vi "NIMS_DF_fir_linfconstr(n, f, mag, ftype, t).vi"(6 "t":enum32{"sym", "antisym", "minphase", "maxphase"}(ring), 8 "ftype":string, 9 "mag":dbl[](array[numeric]), 10 "f":dbl[](array[numeric]), 11 "n":i32) -> (0 "error":i32, 3 "b":dbl[](array[numeric]))   [LabVIEW 2017, in "NI_DigFilter_MathScript.lvlib"]
uses:
  <vilib>/addons/Digital Filter Design/NI_DigFilter_MathScript.lvlib
  <vilib>/addons/Digital Filter Design/_REMEZ.llb/remez_fir filter type.ctl
  <vilib>/addons/Digital Filter Design/NI_DigFilterLicensed.lvlib
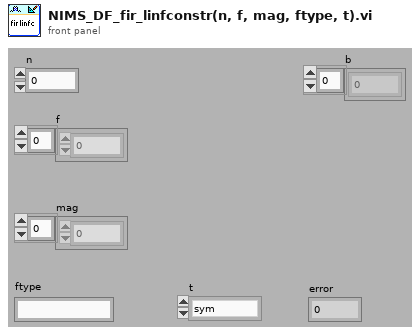
[diagram p1: front panel]
types:
  T1 = typedef "NI_DigFilterLicensed.lvlib/remez_fir filter type.ctl" = enum32{"Symmetric", "Antisymmetric", "Differentiator", "Hilbert", "Minimum Phase", "Maximum Phase"}
  T2 = typedef "NI_DigFilterLicensed.lvlib/DFD Adv Band Spec.ctl" = cluster{"band specification":cluster{"freq":dbl, "amplitude":dbl, "weight":dbl}[], "ripple constraint":dbl}
  T3 = typedef "NI_DigFilterLicensed.lvlib/DFD Filter Obj.ctl" = cluster{"mSRate_Fs":dbl, "mSRate_Version":string, "mSRate_Comments":string, "mSRate_OrgCoef":T4, "mSRate_CurCoef":T4, "mSRate_Quantized?":bool, "mSRate_QCoef":T4, "mSRate_QSettings":T6[], "mSRate_Order":i32, "mSRate_Scaling":cluster{"mSRate_ScaleByPowerOf2?":bool, "mSRate_ScaleType":T8}}
  T4 = typedef "NI_DigFilterLicensed.lvlib/DFD Filter Coef.ctl" = cluster{"type":T5, "gain":dbl, "coef a (k)":dbl[], "coef b (v)":dbl[]}
  T5 = typedef "NI_DigFilterLicensed.lvlib/DFD Filter Structure Type Selector.ctl" = enum16{"Undefined", "FIR Direct Form", "FIR Direct Form Transposed", "FIR Symmetric", "FIR Antisymmetric", "IIR Direct Form I", "IIR Direct Form I Transposed", "IIR Direct Form II", "IIR Direct Form II Transposed", "IIR Cascaded Second Order Sections Form I", "IIR Cascaded Second Order Sections Form I Transposed", "IIR Cascaded Second Order Sections Form II", "IIR Cascaded Second Order Sections Form II Transposed", "Lattice Allpass (basic sections)", "Lattice Allpass (one multiplier sections)", "Lattice Allpass (normalized sections)", "Lattice AR (basic sections)", "Lattice AR (one multiplier sections)", "Lattice AR (normalized sections)", "Lattice MA (minimum phase)", "Lattice MA (maximum phase)", "Lattice ARMA (basic sections)", "Lattice ARMA (one multiplier sections)", "Lattice ARMA (normalized sections)"}
  T6 = typedef "NI_DigFilterLicensed.lvlib/dfd_Internal Quantization Settings.ctl" = cluster{"source":T7, "wl":i16, "iwl":i16, "overflow mode":enum16{"Saturation", "Wrap"}, "rounding mode":enum16{"Nearest", "Truncation"}, "signed?":bool}
  T7 = typedef "NI_DigFilterLicensed.lvlib/dfd_Internal Quantization Srcs.ctl" = u16
  T8 = typedef "NI_DigFilterLicensed.lvlib/DFD Coef Norm Type.ctl" = enum16{"No Norm", "Time Domain 1-Norm", "Time Domain 2-Norm", "Time Domain Inf-Norm"}
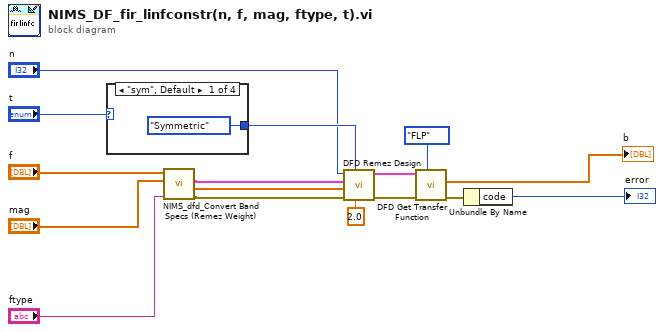
[diagram p0: block diagram]
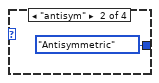
[diagram p2: hidden frame]
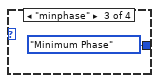
[diagram p3: hidden frame]
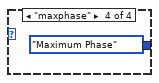
[diagram p4: hidden frame]
diagram:
  n1 = case shown="\"sym\", Default" "t" {
    tunnel: [remez_fir_filter_type."Symmetric" ("filter type") remez_fir_filter_type."Antisymmetric" ("filter type") remez_fir_filter_type."Minimum Phase" ("filter type") remez_fir_filter_type."Maximum Phase" ("filter type")] -> w9
    frame "sym", Default {
    }
    frame "antisym" {
    }
    frame "minphase" {
    }
    frame "maxphase" {
    }
  }
  n2 = call <vilib>:"NIMS_dfd_Convert Band Specs (Remez Weight).vi"("s"="ftype", "A"="mag", "F"="f") -> ("error out"=w3:errorcluster, "freqs of exact gain [Hz]"=w2:dbl[], "band specs"=w4:T2[])  [unwired: 1 in, 5 out]
  n3 = call <vilib>:"DFD Remez Design.vi"("fs [Hz]"=2.0, "filter type"=w9, "error in (no error)"=w3, "freqs of exact gain [Hz]"=w2, "band specs"=w4, "order"="n") -> ("error out"=w14:errorcluster, "filter out"=w15:T3)  [unwired: 1 in, 3 out]
  n4 = call <vilib>:"DFD Get Transfer Function.vi"("type (FLP)"=enum16{"FLP", "FXP"}."FLP", "error in (no error)"=w14, "filter in"=w15) -> ("error out"=w11:errorcluster, "numerator"=→"b":dbl[])  [unwired: 7 out]
  n5 = Unbundle By Name(w11) -> ("code"=→"error":i32)
